vi "VI Tree.vi"   [LabVIEW 2012, in "Quantum Composers 9000 Series.lvlib"]
doc: "This is the instrument driver for the Quantum Composers 9000 Series <Pulse Generator>. The VI Tree displays all the user-callable VIs of the instrument driver in an organized table."
uses:
  <instrlib>/Quantum Composers 9000 Series/Quantum Composers 9000 Series.lvlib
  <instrlib>/Quantum Composers 9000 Series/Public/Action-Status/Query Chan Parameters (Input).vi
  <instrlib>/Quantum Composers 9000 Series/Public/Action-Status/Query Chan Parameters (Output).vi
  <instrlib>/Quantum Composers 9000 Series/Public/Configure/Configure Chan Mode (Normal).vi
  <instrlib>/Quantum Composers 9000 Series/Public/Configure/Configure Sys (To) Mode (Normal).vi
  <instrlib>/Quantum Composers 9000 Series/Public/Action-Status/Query Sys (To) Parameters (Input).vi
  <instrlib>/Quantum Composers 9000 Series/Public/Action-Status/Query Chan Parameters (Mode).vi
  <instrlib>/Quantum Composers 9000 Series/Public/Action-Status/Query Sys (To) Parameters (Mode).vi
panel:
  # "SEE DIAGRAM\nFOR VI TREE."
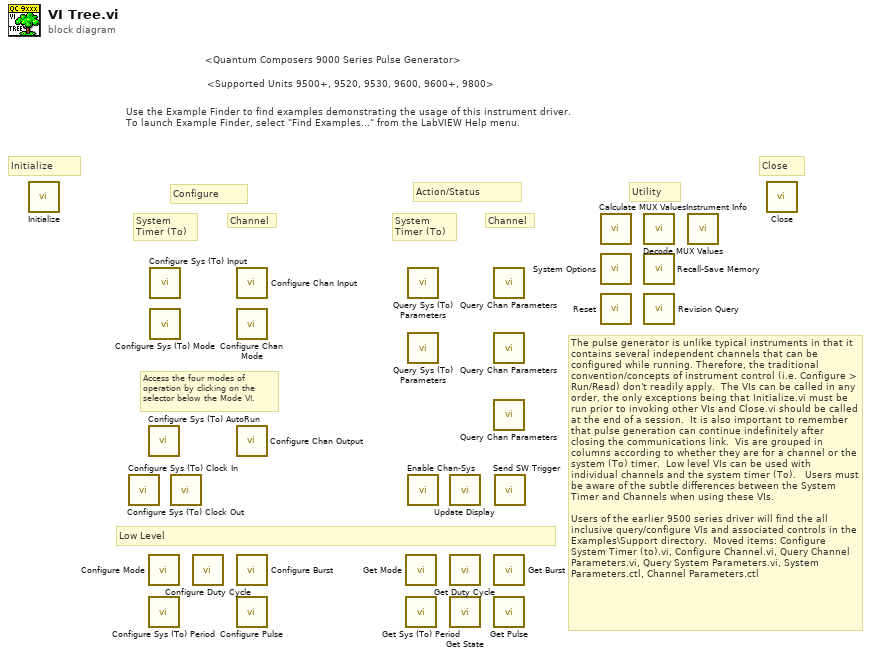
[diagram p0: block diagram]
diagram:
  # "<Supported Units 9500+, 9520, 9530, 9600, 9600+, 9800>"
  # "The pulse generator is unlike typical instruments in that it contains several independent channels that can be configured while running. Therefore, the traditional convention/concepts of instrument control (i.e. Configure > Run/Read) don't readily apply.  The VIs can be called in any order, the only exceptions being that Initialize.vi must be run prior to invoking other VIs and Close.vi should be called at the end of a session.  It is also important to remember that pulse generation can continue indefinitely after closing the communications link.  Vis are grouped in columns according to whether they are for a channel or the system (To) timer.  Low level VIs can be used with individual channels and the system timer (To).   Users must be aware of the subtle differences between the System Timer and Channels when using these VIs. \n\nUsers of the earlier 9500 series driver will find the all inclusive query/configure VIs and associated controls in the Examples\\Support directory.  Moved items: Configure System Timer (to).vi, Configure Channel.vi, Query Channel Parameters.vi, Query System Parameters.vi, System Parameters.ctl, Channel Parameters.ctl"
  # "Channel"
  # "System\nTimer (To)"
  # "Access the four modes of\noperation by clicking on the\nselector below the Mode VI."
  # "Channel"
  # "System\nTimer (To)"
  # "Action/Status"
  # "Low Level"
  # "Configure"
  # "Utility"
  # "Close"
  # "Initialize"
  # "<Quantum Composers 9000 Series Pulse Generator>"
  # "Use the Example Finder to find examples demonstrating the usage of this instrument driver.\nTo launch Example Finder, select \"Find Examples...\" from the LabVIEW Help menu."
  n1 = call <instrlib>:"Initialize.vi"() -> ()  [unwired: 10 in, 2 out]
  n2 = call <instrlib>:"Configure Sys (To) Clock In.vi"() -> ()  [unwired: 10 in, 2 out]
  n3 = call <instrlib>:"Configure Sys (To) AutoRun.vi"() -> ()  [unwired: 10 in, 2 out]
  n4 = call <instrlib>:"Configure Mode.vi"() -> ()  [unwired: 10 in, 2 out]
  n5 = call <instrlib>:"Configure Sys (To) Period.vi"() -> ()  [unwired: 10 in, 2 out]
  n6 = call <instrlib>:"Configure Sys (To) Input.vi"() -> ()  [unwired: 10 in, 2 out]
  n7 = call-poly <instrlib>:"Configure Sys (To) Mode.vi"() -> ()  [unwired: 10 in, 2 out]
  n8 = call <instrlib>:"Configure Sys (To) Clock Out.vi"() -> ()  [unwired: 10 in, 2 out]
  n9 = call <instrlib>:"Configure Duty Cycle.vi"() -> ()  [unwired: 10 in, 2 out]
  n10 = call <instrlib>:"Configure Chan Input.vi"() -> ()  [unwired: 10 in, 2 out]
  n11 = call-poly <instrlib>:"Configure Chan Mode.vi"() -> ()  [unwired: 10 in, 2 out]
  n12 = call <instrlib>:"Configure Chan Output.vi"() -> ()  [unwired: 10 in, 2 out]
  n13 = call <instrlib>:"Configure Burst.vi"() -> ()  [unwired: 10 in, 2 out]
  n14 = call <instrlib>:"Configure Pulse.vi"() -> ()  [unwired: 10 in, 2 out]
  n15 = call <instrlib>:"Get Mode.vi"() -> ()  [unwired: 9 in, 3 out]
  n16 = call <instrlib>:"Get Sys (To) Period.vi"() -> ()  [unwired: 9 in, 3 out]
  n17 = call-poly <instrlib>:"Query Sys (To) Parameters.vi"() -> ()  [unwired: 9 in, 3 out]
  n18 = call-poly <instrlib>:"Query Sys (To) Parameters.vi"() -> ()  [unwired: 9 in, 3 out]
  n19 = call <instrlib>:"Enable Chan-Sys.vi"() -> ()  [unwired: 10 in, 2 out]
  n20 = call <instrlib>:"Update Display.vi"() -> ()  [unwired: 10 in, 2 out]
  n21 = call <instrlib>:"Get Duty Cycle.vi"() -> ()  [unwired: 8 in, 4 out]
  n22 = call <instrlib>:"Get State.vi"() -> ()  [unwired: 9 in, 3 out]
  n23 = call-poly <instrlib>:"Query Chan Parameters.vi"() -> ()  [unwired: 9 in, 3 out]
  n24 = call-poly <instrlib>:"Query Chan Parameters.vi"() -> ()  [unwired: 9 in, 3 out]
  n25 = call-poly <instrlib>:"Query Chan Parameters.vi"() -> ()  [unwired: 9 in, 3 out]
  n26 = call <instrlib>:"Get Burst.vi"() -> ()  [unwired: 9 in, 3 out]
  n27 = call <instrlib>:"Get Pulse.vi"() -> ()  [unwired: 7 in, 5 out]
  n28 = call <instrlib>:"Send SW Trigger.vi"() -> ()  [unwired: 10 in, 2 out]
  n29 = call <instrlib>:"Calculate MUX Values.vi"() -> ()  [unwired: 9 in, 3 out]
  n30 = call <instrlib>:"System Options.vi"() -> ()  [unwired: 10 in, 2 out]
  n31 = call <instrlib>:"Reset.vi"() -> ()  [unwired: 10 in, 2 out]
  n32 = call <instrlib>:"Decode MUX Values.vi"() -> ()  [unwired: 9 in, 3 out]
  n33 = call <instrlib>:"Recall-Save Memory.vi"() -> ()  [unwired: 10 in, 2 out]
  n34 = call <instrlib>:"Revision Query.vi"() -> ()  [unwired: 4 in, 8 out]
  n35 = call <instrlib>:"Instrument Info.vi"() -> ()  [unwired: 8 in, 4 out]
  n36 = call <instrlib>:"Close.vi"() -> ()  [unwired: 11 in, 1 out]
